vi "Arduino rentel.vi"() -> ()   [LabVIEW 2013]
uses:
  <vilib>/Instr/_visa.llb/VISA Configure Serial Port (Instr).vi
  <vilib>/picture/3D Picture Control/Object/Create Object (name).vi
  <vilib>/picture/3D Picture Control/NI_3D Picture Control.lvlib
panel:
  out "Inclinación":refnum<vi>(3d-picture)
  out "FRASE COMPLETA":string
  out "Aceleración Y":string
  out "Aceleración Z":string
  out "Aceleración X":string
  out "Angulo Z":string
  out "Angulo Y":string
  out "Angulo X":string
  out "Cº":string
  out "Temp ambiente":dbl(slide) scale=0.0..100.0
  out "Temp motor 2":dbl(slide) scale=0.0..100.0
  out "Trabajo":dbl(knob) scale=0.0..30000.0
  out "Amperaje":dbl(knob) scale=0.0..200.0
  out "Voltaje":dbl(knob) scale=0.0..150.0
  out "Watios":i32[](graph)
  out "Amperaje":i32[](graph)
  out "Voltaje":i32[](graph)
  out "Tiempo pasado":string
  out "Rpm":dbl(knob) scale=0.0..4000.0
  out "Temp motor":dbl(slide) scale=0.0..100.0
  out "Rpm":string
  out "Cº":string
  out "W":string
  out "V":string
  out "A":string
  in  "Parar":bool
  in  "On":bool
  in  "flow control":u16(ring) items=["None"=0, "XON/XOFF"=1, "RTS/CTS"=2, "DTR/DSR"=4]
  in  "stop bits":u16(ring)=10 items=["1.0"=10, "1.5"=15, "2.0"=20]
  in  "parity":u16(ring) items=["None", "Odd", "Even", "Mark", "Space"]
  in  "data bits":u16=8 min=5 max=8 step=1
  in  "VISA resource name":refnum<visa-resource-name>="COM1"
  in  "baud rate":u32=9600
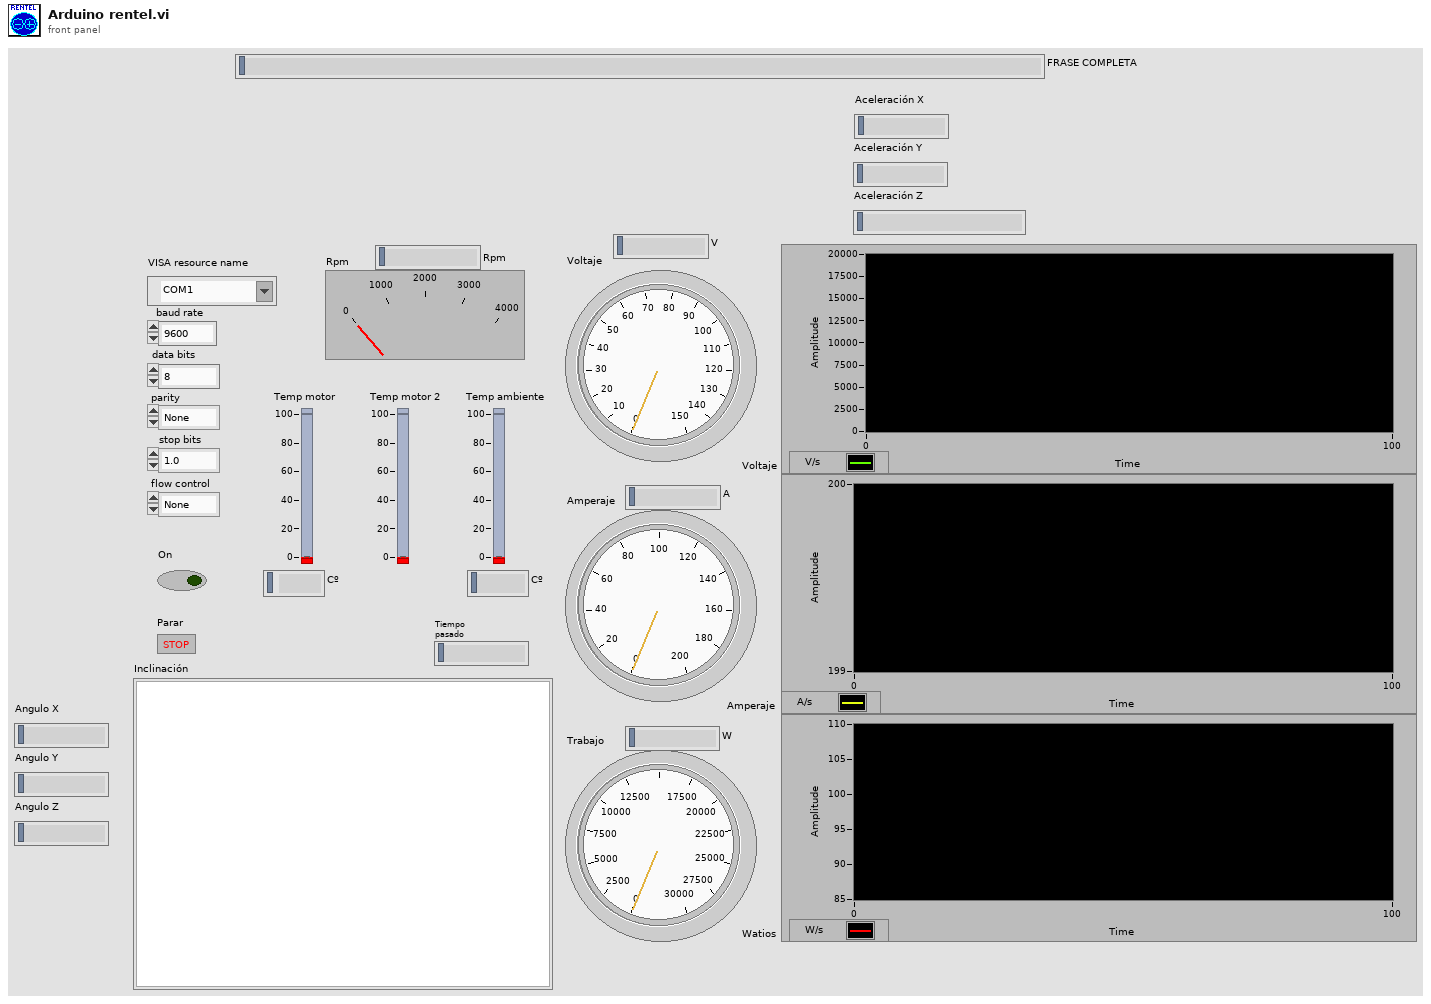
[diagram p1: front panel]
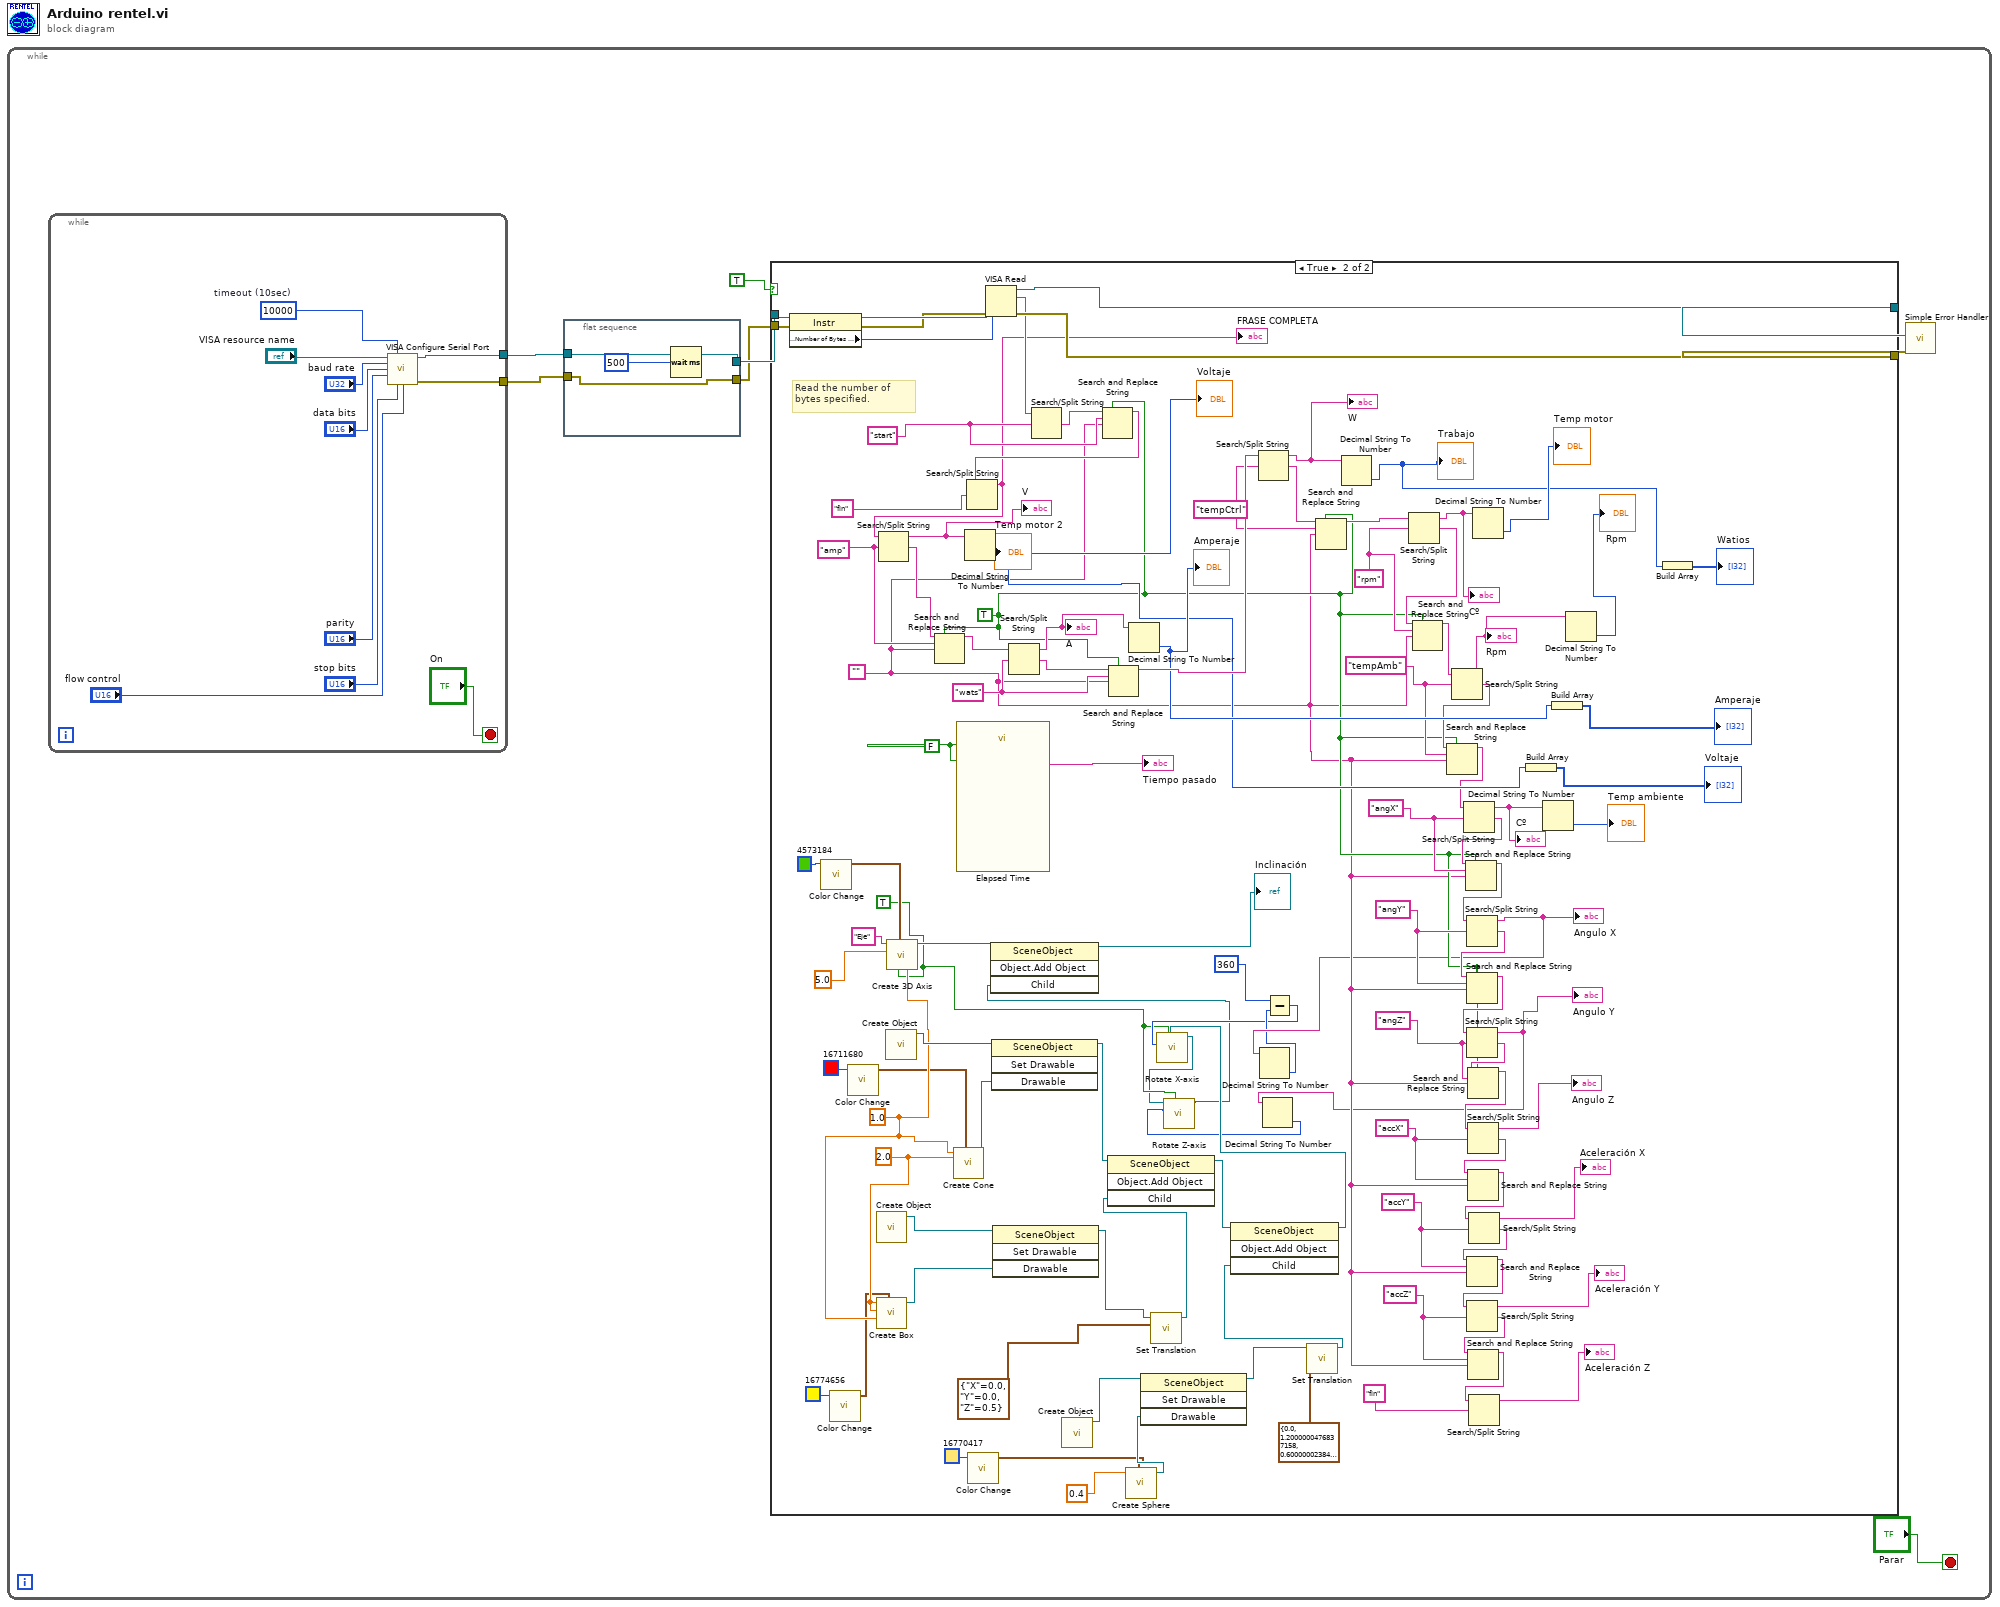
[diagram p0: block diagram]
diagram:
  n1 = while {
    stop <- "Parar" stop-if-true
    n2 = while {
      tunnel: [w122] -> w8
      tunnel: [w121] -> w7
      stop <- "On" stop-if-true
      w126 = u32 10000  # timeout (10sec)
      n3 = call-poly "VISA Configure Serial Port"("VISA resource name"="VISA resource name", "timeout (10sec)"=w126, "baud rate (9600)"="baud rate", "data bits (8)"="data bits", "parity (0:none)"="parity", "stop bits (10: 1 bit)"="stop bits", "flow control (0:none)"="flow control") -> ("VISA resource name out"=w122:refnum<visa-resource-name>, "error out"=w121:errorcluster)  [unwired: 2 in, 5 out]
    }
    n4 = flat-sequence {
      tunnel: w8 -> [w130]
      tunnel: w7 -> [w131]
      tunnel: [w131] -> w3
      tunnel: [w130] -> w4
      frame #0 {
        n5 = Wait (ms)(milliseconds to wait=500) -> ()  [unwired: 1 out]
      }
    }
    n6 = case shown="True" TRUE {
      tunnel: w4 -> [w10 w114]
      tunnel: w3 -> [w9 w113]
      tunnel: [w9 w118] -> w6
      tunnel: [w10 w115] -> w5
      frame False {
      }
      frame True {
        w42 = 2.0
        w36 = 1.0
        w16 = TRUE
        w61 = "accY"
        w58 = "accZ"
        w65 = "accX"
        w70 = "angZ"
        w73 = "angY"
        w76 = "angX"
        w81 = "tempAmb"
        w88 = FALSE
        w92 = "start"
        w99 = "rpm"
        w103 = "tempCtrl"
        w106 = "wats"
        w69 = TRUE
        w52 = ""
        w111 = "amp"
        # "Read the number of bytes specified."
        n7 = property class="Instr"(reference=w114, error in=w113) -> (reference out=w119:refnum<visa-resource-name>, error out=w116:errorcluster, "Serial Settings:Number of Bytes at Serial Port"=w117:u32)
        n8 = call <vilib>:"Color Change.vi"("Color"=u32 4573184) -> ("RGBA"=w33:cluster{"R":sgl, "G":sgl, "B":sgl, "A":sgl})  [unwired: 10 in]
        n9 = call <vilib>:"Color Change.vi"("Color"=u32 16774656) -> ("RGBA"=w31:cluster{"R":sgl, "G":sgl, "B":sgl, "A":sgl})  [unwired: 10 in]
        n10 = call <vilib>:"Color Change.vi"("Color"=u32 16711680) -> ("RGBA"=w30:cluster{"R":sgl, "G":sgl, "B":sgl, "A":sgl})  [unwired: 10 in]
        n11 = call-poly <vilib>:"Create Object.vi"() -> ("Scene:New Object"=w46:refnum<vi>)  [unwired: 10 in, 1 out]
        n12 = call <vilib>:"Create Box.vi"("Color"=w31, "Length Z"=w36, "Length Y"=w42, "Length X"=w42) -> ("New Box Refnum"=w45:refnum<vi>)  [unwired: 6 in, 1 out]
        n13 = call-poly <vilib>:"Create Object.vi"() -> ("Scene:New Object"=w49:refnum<vi>)  [unwired: 10 in, 1 out]
        n14 = call <vilib>:"Create 3D Axis.vi"("Character Size"=w36, "Axis label?"=w16, "Color"=w33, "Length"=5.0, "Name"="Eje") -> ("New Object Refnum"=w51:refnum<vi>)  [unwired: 5 in, 1 out]
        n15 = call <vilib>:"Create Cone.vi"("Color"=w30, "Radius"=w42, "Height"=w36) -> ("New Cone Refnum"=w48:refnum<vi>)  [unwired: 7 in, 1 out]
        n16 = call "Elapsed Time"("Reset"=w88, "Auto Reset"=w88) -> ("Elapsed Time Text"=→"Tiempo pasado":string)  [unwired: 10 in, 7 out]
        n17 = call <vilib>:"Color Change.vi"("Color"=u32 16770417) -> ("RGBA"=w17:cluster{"R":sgl, "G":sgl, "B":sgl, "A":sgl})  [unwired: 10 in]
        n18 = VISA Read(VISA resource name=w119, byte count=w117, error in (no error)=w116) -> (VISA resource name out=w115:refnum<visa-resource-name>, read buffer=w87:string, error out=w118:errorcluster)  [unwired: 1 out]
        n19 = invoke class="SceneObject" method="Set Drawable"(reference=w49, "Drawable"=w48) -> (reference out=w47:refnum<vi>)  [unwired: 2 in, 3 out]
        n20 = invoke class="SceneObject" method="Set Drawable"(reference=w46, "Drawable"=w45) -> (reference out=w44:refnum<vi>)  [unwired: 2 in, 3 out]
        n21 = Search/Split String(string=w87, search string/char (-)=w92) -> (match + rest of string=w94:string)  [unwired: 1 in, 2 out]
        n22 = call-poly <vilib>:"Create Object.vi"() -> ("Scene:New Object"=w26:refnum<vi>)  [unwired: 10 in, 1 out]
        n23 = Search and Replace String(replace all?=w69, input string=w94, search string=w92, replace string=w52) -> (result string=w93:string)  [unwired: 4 in, 3 out]
        n24 = Search/Split String(string=w93, search string/char (-)="fin") -> (substring before match=w53:string)  [unwired: 1 in, 2 out]
        "FRASE COMPLETA" <- w53
        n25 = Search/Split String(string=w53, search string/char (-)=w111) -> (substring before match=w112:string, match + rest of string=w110:string)  [unwired: 1 in, 1 out]
        "V" <- w112
        n26 = Search and Replace String(replace all?=w69, input string=w110, search string=w111, replace string=w52) -> (result string=w109:string)  [unwired: 4 in, 3 out]
        n27 = Decimal String To Number(string=w112) -> (number=w84:i32)  [unwired: 2 in, 1 out]
        "Voltaje" <- w84
        n28 = Search/Split String(string=w109, search string/char (-)=w106) -> (substring before match=w108:string, match + rest of string=w107:string)  [unwired: 1 in, 1 out]
        "A" <- w108
        n29 = Search and Replace String(replace all?=w69, input string=w107, search string=w106, replace string=w52) -> (result string=w105:string)  [unwired: 4 in, 3 out]
        n30 = call <vilib>:"Create Sphere.vi"("Color"=w17, "Radius"=0.4) -> ("New Sphere Refnum"=w25:refnum<vi>)  [unwired: 8 in, 1 out]
        n31 = Decimal String To Number(string=w108) -> (number=w85:i32)  [unwired: 2 in, 1 out]
        "Amperaje" <- w85
        n32 = invoke class="SceneObject" method="Set Drawable"(reference=w26, "Drawable"=w25) -> (reference out=w24:refnum<vi>)  [unwired: 2 in, 3 out]
        n33 = call <vilib>:"Set Translation.vi"("Translation"=cluster{"X":sgl, "Y":sgl, "Z":sgl} {"X"=0.0, "Y"=0.0, "Z"=0.5}, "Scene Object"=w44) -> ("Translated Object"=w43:refnum<vi>)  [unwired: 8 in, 1 out]
        n34 = invoke class="SceneObject" method="Object.Add Object"(reference=w47, "Child"=w43) -> (reference out=w20:refnum<vi>)  [unwired: 2 in, 3 out]
        n35 = Search/Split String(string=w105, search string/char (-)=w103) -> (substring before match=w101:string, match + rest of string=w104:string)  [unwired: 1 in, 1 out]
        "W" <- w101
        n36 = call <vilib>:"Set Translation.vi"("Translation"=cluster{"X":sgl, "Y":sgl, "Z":sgl} {"X"=0.0, "Y"=1.2, "Z"=0.6}, "Scene Object"=w24) -> ("Translated Object"=w21:refnum<vi>)  [unwired: 8 in, 1 out]
        n37 = invoke class="SceneObject" method="Object.Add Object"(reference=w20, "Child"=w21) -> (reference out=w19:refnum<vi>)  [unwired: 2 in, 3 out]
        n38 = Search and Replace String(replace all?=w69, input string=w104, search string=w103, replace string=w52) -> (result string=w102:string)  [unwired: 4 in, 3 out]
        n39 = Decimal String To Number(string=w101) -> (number=w83:i32)  [unwired: 2 in, 1 out]
        "Trabajo" <- w83
        n40 = Search/Split String(string=w102, search string/char (-)=w99) -> (substring before match=w100:string, match + rest of string=w98:string)  [unwired: 1 in, 1 out]
        "Cº" <- w100
        n41 = Search and Replace String(replace all?=w69, input string=w98, search string=w99, replace string=w52) -> (result string=w97:string)  [unwired: 4 in, 3 out]
        n42 = Search/Split String(string=w97, search string/char (-)=w81) -> (substring before match=w96:string, match + rest of string=w82:string)  [unwired: 1 in, 1 out]
        "Rpm" <- w96
        n43 = Search and Replace String(replace all?=w69, input string=w82, search string=w81, replace string=w52) -> (result string=w80:string)  [unwired: 4 in, 3 out]
        n44 = Search/Split String(string=w80, search string/char (-)=w76) -> (substring before match=w78:string, match + rest of string=w77:string)  [unwired: 1 in, 1 out]
        "Cº" <- w78
        n45 = Search and Replace String(replace all?=w69, input string=w77, search string=w76, replace string=w52) -> (result string=w75:string)  [unwired: 4 in, 3 out]
        n46 = Search/Split String(string=w75, search string/char (-)=w73) -> (substring before match=w39:string, match + rest of string=w74:string)  [unwired: 1 in, 1 out]
        "Angulo X" <- w39
        n47 = Decimal String To Number(string=w39) -> (number=w28:i32)  [unwired: 2 in, 1 out]
        n48 = Subtract(x=360, y=w28) -> (x-y=w27:i32)
        n49 = call <vilib>:"Rotate X-axis.vi"("Relative?"=w16, "angle"=w27, "Scene Object In"=w19) -> ("Scene Object Out"=w15:refnum<vi>)  [unwired: 7 in, 1 out]
        n50 = Search and Replace String(replace all?=w69, input string=w74, search string=w73, replace string=w52) -> (result string=w72:string)  [unwired: 4 in, 3 out]
        n51 = Search/Split String(string=w72, search string/char (-)=w70) -> (substring before match=w38:string, match + rest of string=w71:string)  [unwired: 1 in, 1 out]
        "Angulo Y" <- w38
        n52 = Decimal String To Number(string=w38) -> (number=w14:i32)  [unwired: 2 in, 1 out]
        n53 = call <vilib>:"Rotate Z-axis.vi"("Relative?"=w16, "angle"=w14, "Scene Object In"=w15) -> ("Scene Object Out"=w13:refnum<vi>)  [unwired: 7 in, 1 out]
        n54 = invoke class="SceneObject" method="Object.Add Object"(reference=w51, "Child"=w13) -> (reference out=→"Inclinación":refnum<vi>)  [unwired: 2 in, 3 out]
        n55 = Search and Replace String(replace all?=w69, input string=w71, search string=w70, replace string=w52) -> (result string=w68:string)  [unwired: 4 in, 3 out]
        n56 = Search/Split String(string=w68, search string/char (-)=w65) -> (substring before match=→"Angulo Z":string, match + rest of string=w66:string)  [unwired: 1 in, 1 out]
        n57 = Search and Replace String(input string=w66, search string=w65, replace string=w52) -> (result string=w64:string)  [unwired: 5 in, 3 out]
        n58 = Search/Split String(string=w64, search string/char (-)=w61) -> (substring before match=→"Aceleración X":string, match + rest of string=w62:string)  [unwired: 1 in, 1 out]
        n59 = Search and Replace String(input string=w62, search string=w61, replace string=w52) -> (result string=w60:string)  [unwired: 5 in, 3 out]
        n60 = Search/Split String(string=w60, search string/char (-)=w58) -> (substring before match=→"Aceleración Y":string, match + rest of string=w57:string)  [unwired: 1 in, 1 out]
        n61 = Search and Replace String(input string=w57, search string=w58, replace string=w52) -> (result string=w56:string)  [unwired: 5 in, 3 out]
        n62 = Search/Split String(string=w56, search string/char (-)="fin") -> (substring before match=→"Aceleración Z":string)  [unwired: 1 in, 2 out]
        n63 = Decimal String To Number(string=w100) -> (number=→"Temp motor":i32)  [unwired: 2 in, 1 out]
        n64 = Build Array(w84) -> (→"Voltaje":i32[])
        n65 = Decimal String To Number(string=w78) -> (number=→"Temp ambiente":i32)  [unwired: 2 in, 1 out]
        n66 = Build Array(w85) -> (→"Amperaje":i32[])
        n67 = Decimal String To Number(string=w96) -> (number=→"Rpm":i32)  [unwired: 2 in, 1 out]
        n68 = Build Array(w83) -> (→"Watios":i32[])
      }
    }
    n69 = call <vilib>:"Simple Error Handler.vi"("error source (\" \")"=w5, "error in (no error)"=w6) -> ()  [unwired: 1 in, 7 out]
  }
